vi "[RT] Array_And_Size.vi"(2 "Select":enum16{"READ", "WRITE"}(ring), 3 "Size":i32, 4 "Data In":dbl[](array[numeric])) -> (0 "Size":i32, 1 "Data Out":dbl[](array[numeric]))   [LabVIEW 2018]
panel:
  out "error out":errorcluster
  in  "error in":errorcluster
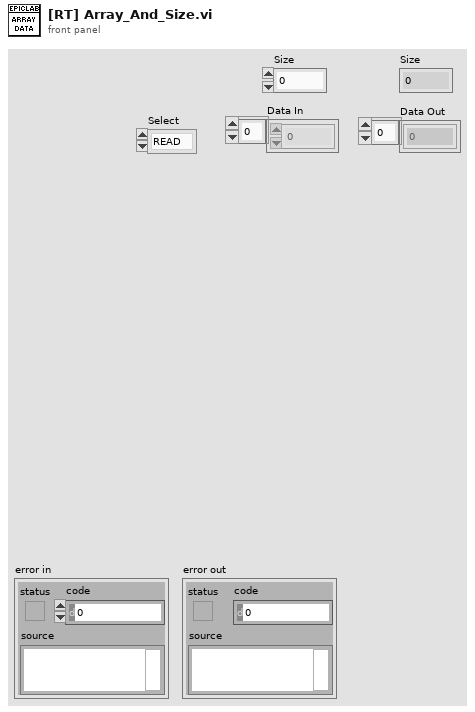
[diagram p1: front panel]
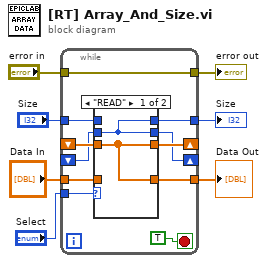
[diagram p0: block diagram]
diagram:
  n1 = while {
    tunnel: "Select" -> [w18]
    tunnel: [w17] -> w5
    tunnel: "error in" -> [w17]
    tunnel: [w16] -> w3
    shift-right: [w15] -> _
    shift-left: _ -> [w14]
    tunnel: "Data In" -> [w13]
    shift-right: [w11] -> _
    shift-left: _ -> [w8]
    tunnel: [w10] -> w2
    tunnel: "Size" -> [w9]
    stop <- TRUE stop-if-true
    n2 = case shown="\"READ\"" w18 {
      tunnel: w14 -> [w20 _]
      tunnel: [w20 w22] -> w16
      tunnel: [w20 w22] -> w15
      tunnel: w13 -> [_ w22]
      tunnel: w9 -> [_ w21]
      tunnel: [w19 w21] -> w11
      tunnel: [w19 w21] -> w10
      tunnel: w8 -> [w19 _]
      frame "READ" {
      }
      frame "WRITE" {
      }
    }
  }
  "error out" <- w5
  "Data Out" <- w3
  "Size" <- w2
